vi "Is_Playbacked.vi"(0 "Index":i32, 5 "Playback?":bool, 9 "Event_Data":dbl) -> (4 "Is_Playback":bool)   [LabVIEW 2021]
doc: "Used to check if already playbacked"
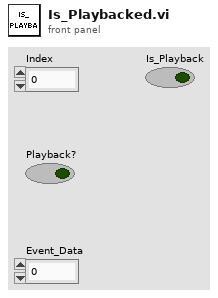
[diagram p1: front panel]
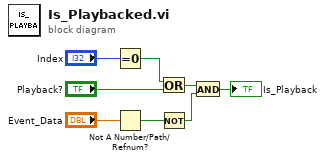
[diagram p0: block diagram]
diagram:
  n1 = Equal To 0?(x="Index") -> (x = 0?=w3:bool)
  n2 = Not A Number/Path/Refnum?(number/path/refnum="Event_Data") -> (NaN/Path/Refnum?=w6:bool)
  n3 = Or(x=w3, y="Playback?") -> (x .or. y?=w2:bool)
  n4 = Not(x=w6) -> (.not. x?=w8:bool)
  n5 = And(x=w2, y=w8) -> (x .and. y?=→"Is_Playback":bool)
